vi "S2C_Access_Column1Select.vi"(8 "Error In":errorcluster, 11 "Table":string) -> (0 "Error Out":errorcluster)   [LabVIEW 2015]
uses:
  S2C_Access_Globals.vi
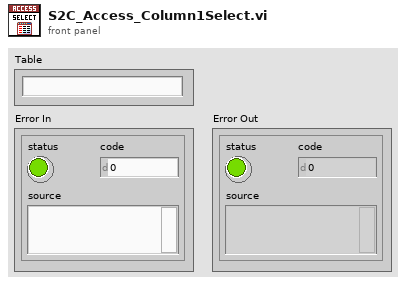
[diagram p1: front panel]
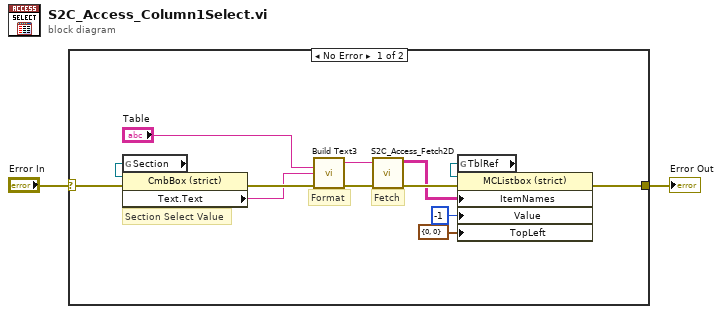
[diagram p0: block diagram]
diagram:
  n1 = case shown="No Error" "Error In" {
    selector: "Error In" -> [w4 w16]
    tunnel: [w3 w16] -> w1
    frame No Error {
      # "Format"
      # "Fetch"
      # "Section Select Value"
      n2 = global read "S2C_Access_Globals.vi" "Section"() -> (w14:refnum<vi>)
      n3 = property class="CmbBox (strict)"(reference=w14, error in=w4) -> (error out=w11:errorcluster, "Text.Text"=w5:string)  [unwired: 1 out]
      n4 = call "Build Text3"("Table"="Table", "Section"=w5, "error in (no error)"=w11) -> ("Result"=w9:string, "error out"=w10:errorcluster)  [unwired: 11 in]
      n5 = call "S2C_Access_Fetch2D.vi"("Error In"=w10, "Query"=w9) -> ("Error Out"=w13:errorcluster, "Data"=w12:string[][])  [unwired: 8 in]
      n6 = global read "S2C_Access_Globals.vi" "TblRef"() -> (w15:refnum<vi>)
      n7 = property class="MCListbox (strict)"(reference=w15, error in=w13, "ItemNames"=w12, "Value"=-1, "TopLeft"=cluster{"Row":u32, "Column":u32} {"Row"=0, "Column"=0} ("Top Left Visible Cell")) -> (error out=w3:errorcluster)  [unwired: 1 out]
    }
    frame Error {
    }
  }
  "Error Out" <- w1
